vi "MAX-SP-AddResultChannel.vi"(8 "Error In":errorcluster, 10 "CD Settings in":T1 {"CD Task Dependency Ref" format="%.0x"; "CD Task Dependency" format="%.0x"}, 11 "Device Ref in":T2=18446744073709551615 format="%.0x") -> (0 "Error Out":errorcluster, 3 "Device Ref Out":T2=18446744073709551615 format="%.0x")   [LabVIEW 2017, in "Waveform-Processing-Custom-Device Shared.lvlib" / "Max_SP.lvlib"]
doc: "This application Adds all of the Child \"Maximum\" output channels found when the \"Add\" option is selected"
uses:
  Max_SP.lvlib
  <vilib>/NI Veristand/Custom Device API/Custom Device Item Ref.ctl
  Custom Device Settings.ctl
  <vilib>/NI Veristand/Custom Device API/Custom Device Channel.ctl
  <vilib>/NI Veristand/Custom Device API/Custom Device Channel Type.ctl
  NationalInstruments.VeriStand.SystemStorage
  Constants.vi
  <vilib>/NI Veristand/Custom Device API/Get Item Property (Dependent Node Pointer).vi
  <vilib>/NI Veristand/Custom Device API/Set Item Property (Dependent Node Pointer).vi
  System Explorer/Waveform-Processing-Custom-Device System Explorer.lvlib
  <vilib>/NI Veristand/Custom Device API/Custom Device API.lvlib
  Waveform-Processing-Custom-Device Shared.lvlib
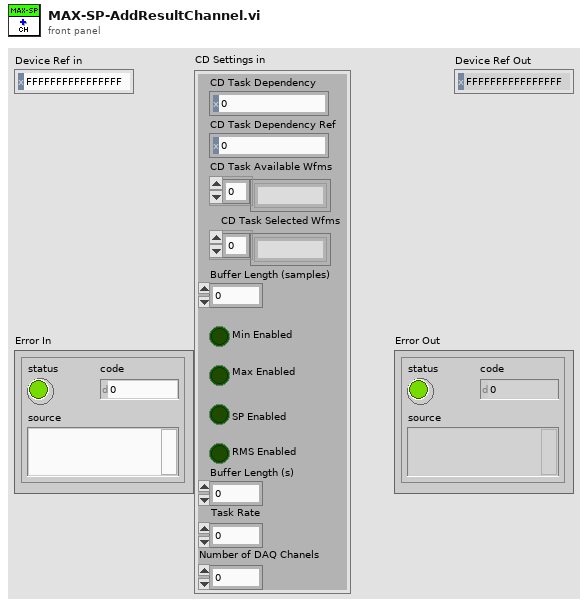
[diagram p1: front panel]
types:
  T1 = typedef "Waveform-Processing-Custom-Device Shared.lvlib/Custom Device Settings.ctl" = cluster{"CD Task Dependency":T2, "CD Task Dependency Ref":T2, "CD Task Available Wfms":string[], "CD Task Selected Wfms":string[], "Buffer Length (samples)":u32, "Min Enabled":bool, "Max Enabled ":bool, "SP Enabled":bool, "RMS Enabled":bool, "Buffer Length (s)":dbl, "Task Rate":dbl, "Number of DAQ Chanels":u32}
  T2 = typedef "Custom Device API.lvlib/Custom Device Item Ref.ctl" = u64
  T3 = typedef "Custom Device API.lvlib/Custom Device Channel Type.ctl" = enum16{"Input", "Output"}
  T4 = typedef "Custom Device API.lvlib/Custom Device Channel.ctl" = cluster{"Type":T3, "Units":string, "Default Value":dbl, "Faultable":bool, "Scalable":bool}
  T5 = cluster{"Waveform Name":string, "Units":string}[]
  T6 = typedef "Custom Device API.lvlib/Custom Device Pointer.ctl" = refnum<k24>
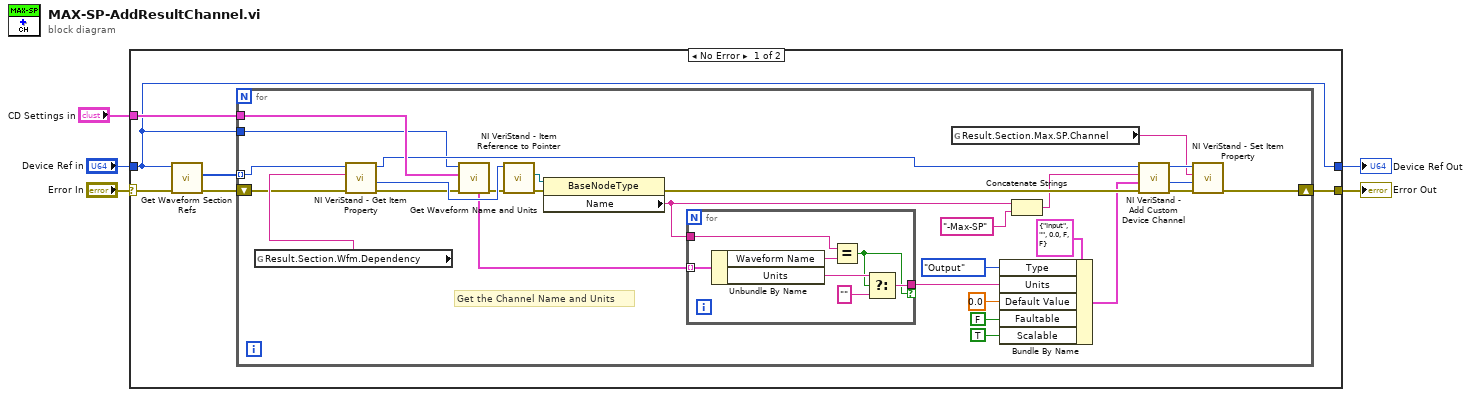
[diagram p0: block diagram]
diagram:
  n1 = case shown="No Error" "Error In" {
    selector: "Error In" -> [w11 w48]
    tunnel: [w10 w48] -> w4
    tunnel: "Device Ref in" -> [w8 w47]
    tunnel: [w8 w47] -> w3
    tunnel: "CD Settings in" -> [w9 _]
    frame No Error {
      n2 = call "Get Waveform Section Refs.vi"("Error in"=w11, "Device Ref in"=w8) -> ("Error out"=w6:errorcluster, "Result Section Refs"=w7:T2[])  [unwired: 7 in, 1 out]
      n3 = for {
        tunnel: w7 -> [w21] mode=indexing
        shift-right: [w33] -> w10
        shift-left: w6 -> [w22]
        tunnel: w9 -> [w19]
        tunnel: w8 -> [w15]
        # "Get the Channel Name and Units"
        n4 = global read "Constants.vi" "Result.Section.Wfm.Dependency"() -> (w29:string)
        n5 = call-poly <vilib>:"NI VeriStand - Get Item Property.vi"("error in (no error)"=w22, "Property Name"=w29, "Item Ref in"=w21) -> ("error out"=w18:errorcluster, "Dependent Node Ref"=w20:T2, "Item Ref out"=w16:T2)  [unwired: 5 in, 1 out]
        n6 = call "Get Waveform Name and Units.vi"("Error In"=w18, "CD Settings"=w19, "CustomDevice Ref"=w15) -> ("Error Out"=w17:errorcluster, "Waveform Channel Name and Units"=w12:T5)  [unwired: 7 in]
        n7 = call <vilib>:"NI VeriStand - Item Reference to Pointer.vi"("error in (no error)"=w17, "Item Ref in"=w20) -> ("error out"=w39:errorcluster, "Node Pointer"=w38:T6)  [unwired: 6 in, 2 out]
        n8 = property class="BaseNodeType"(reference=w38, error in=w39) -> (error out=w36:errorcluster, "Name"=w14:string)  [unwired: 1 out]
        n9 = for {
          tunnel: w12 -> [w45] mode=indexing
          tunnel: w14 -> [w46]
          tunnel: [w42] -> w13 if=w40
          n10 = Unbundle By Name(w45) -> ("Waveform Name"=w44:string, "Units"=w43:string)
          n11 = Equal?(x=w46, y=w44) -> (x = y?=w40:bool)
          n12 = Select(t=w43, s=w40, f="") -> (s? t:f=w42:string)
        }
        n13 = global read "Constants.vi" "Result.Section.Max.SP.Channel"() -> (w31:string)
        n14 = Bundle By Name(cluster=T4 {"Type"=enum."Input", "Units"="", "Default Value"=0.0, "Faultable"=FALSE, "Scalable"=FALSE} ("Channel"), "Type"=Custom_Device_Channel_Type."Output", "Units"=w13, "Default Value"=0.0, "Faultable"=FALSE, "Scalable"=TRUE) -> (w27:T4)
        n15 = Concatenate Strings(w14, "-Max-SP" ("Property Name")) -> (w35:string)
        n16 = call <vilib>:"NI VeriStand - Add Custom Device Channel.vi"("error in (no error)"=w36, "Channel"=w27, "Channel Name"=w35, "Parent Ref in"=w16) -> ("error out"=w34:errorcluster, "Channel Ref"=w30:T2, "Parent Ref out"=w32:T2)  [unwired: 4 in, 1 out]
        n17 = call-poly <vilib>:"NI VeriStand - Set Item Property.vi"("error in (no error)"=w34, "Dependent Node Ref"=w30, "Property Name"=w31, "Item Ref in"=w32) -> ("error out"=w33:errorcluster)  [unwired: 5 in, 2 out]
      }
    }
    frame Error {
    }
  }
  "Error Out" <- w4
  "Device Ref Out" <- w3
